vi "Get Pos Impl.vi"(8 "error in (no error)":errorcluster, 11 "Nikon Ti2 Stage in":refnum<class "Nikon Ti2 Stage.lvclass">) -> (0 "error out":errorcluster, 2 "Stage Position":T1, 3 "Nikon Ti2 Stage out":refnum<class "Nikon Ti2 Stage.lvclass">)   [LabVIEW 2023, in "Nikon Ti2 Stage.lvlib" / "Nikon Ti2 Stage.lvclass"]
uses:
  Nikon Ti2 Stage.lvclass
  Resources/Type Defs/Stage Position.ctl
  Nikon Ti2 Stage.lvclass/Nikon Ti2 Stage.ctl
  Microscope/ti2lv/ti2lv.lvlib
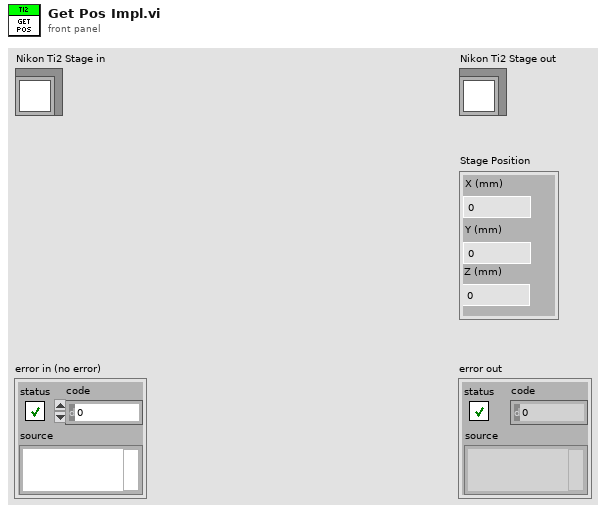
[diagram p1: front panel]
types:
  T1 = typedef "Stage Position.ctl" = cluster{"X (mm)":dbl, "Y (mm)":dbl, "Z (mm)":dbl}
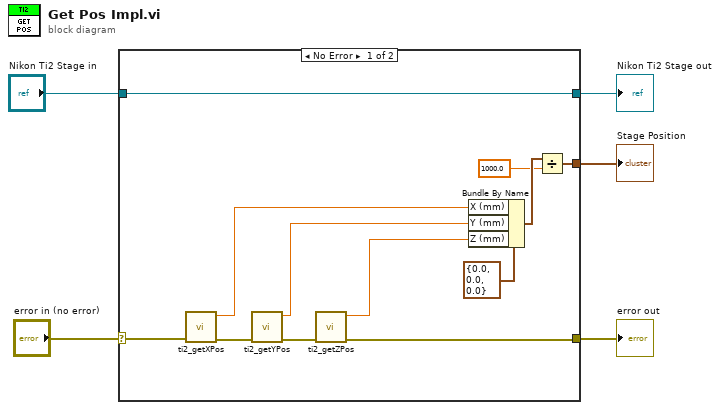
[diagram p0: block diagram]
diagram:
  n1 = case shown="No Error" "error in (no error)" {
    selector: "error in (no error)" -> [w13 w18]
    tunnel: "Nikon Ti2 Stage in" -> [w17 w19]
    tunnel: [w17 w19] -> w4
    tunnel: [w12 w18] -> w2
    tunnel: [w8 _] -> w1
    frame No Error {
      n2 = call "ti2_getXPos.vi"("error in (no error)"=w13) -> ("error out"=w15:errorcluster, "x Position (um)"=w9:dbl)  [unwired: 9 in]
      n3 = call "ti2_getYPos.vi"("error in (no error)"=w15) -> ("error out"=w14:errorcluster, "y Position (um)"=w10:dbl)  [unwired: 9 in]
      n4 = call "ti2_getZPos.vi"("error in (no error)"=w14) -> ("error out"=w12:errorcluster, "z Position (um)"=w11:dbl)  [unwired: 9 in]
      n5 = Bundle By Name(cluster=T1 {"X (mm)"=0.0, "Y (mm)"=0.0, "Z (mm)"=0.0} ("Stage Position 2"), "X (mm)"=w9, "Y (mm)"=w10, "Z (mm)"=w11) -> (w7:T1)
      n6 = Divide(x=w7, y=1000.0) -> (x/y=w8:T1)
    }
    frame Error {
    }
  }
  "error out" <- w2
  "Nikon Ti2 Stage out" <- w4
  "Stage Position" <- w1
